vi "Zasilacz(HP_zas).vi"(8 "error in (no error)":errorcluster, 9 "Source":enum16{"P6V", "P25V"}(ring), 10 "Voltage":dbl, 11 "VISA Refnum in":refnum<visa-resource-name>) -> (0 "error out":errorcluster, 3 "VISA Refnum out":refnum<visa-resource-name>)   [LabVIEW 2020]
uses:
  lib/VirtualLab.lvlibp/VISASimulator/VISALib.lvlib
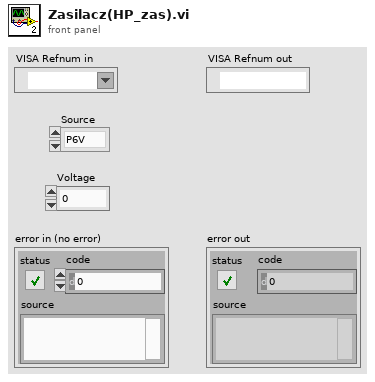
[diagram p1: front panel]
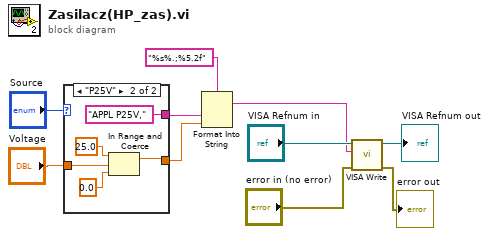
[diagram p0: block diagram]
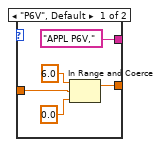
[diagram p2: hidden frame]
diagram:
  n1 = case shown="\"P25V\"" "Source" {
    tunnel: ["APPL P6V," ("write buffer") "APPL P25V," ("write buffer")] -> w5
    tunnel: "Voltage" -> [w12 w16]
    tunnel: [w11 w17] -> w1
    frame "P6V", Default {
      n2 = In Range and Coerce(upper limit=6.0, x=w12, lower limit=0.0) -> (coerced(x)=w11:dbl)  [unwired: 1 out]
    }
    frame "P25V" {
      n3 = In Range and Coerce(upper limit=25.0, x=w16, lower limit=0.0) -> (coerced(x)=w17:dbl)  [unwired: 1 out]
    }
  }
  n4 = Format Into String(format string="%s%.;%5.2f", w5, w1) -> (resulting string=w4:string)  [unwired: 2 in, 1 out]
  n5 = call "VISA Write.vi"("error in (no error)"="error in (no error)", "write buffer"=w4, "VISA resource name"="VISA Refnum in") -> ("error out"=→"error out":errorcluster, "VISA resource name out"=→"VISA Refnum out":refnum<visa-resource-name>)  [unwired: 6 in, 1 out]
